vi "GetVIFolderPath.vi"(8 "error in (no error)":errorcluster, 11 "VI Reference in":refnum<vi>) -> (0 "error out":errorcluster, 3 "VI Folder Path out":path)   [LabVIEW 2015, in "VeriStandTestUtilities.lvlib"]
uses:
  VeriStandTestUtilities.lvlib
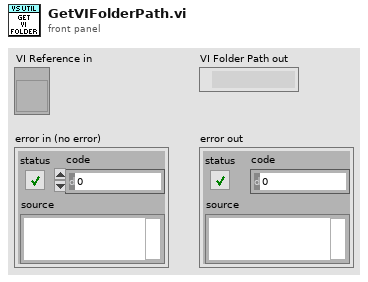
[diagram p1: front panel]
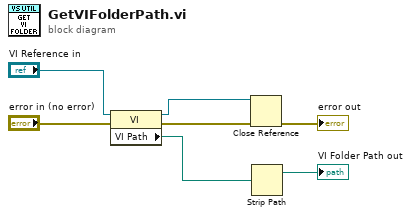
[diagram p0: block diagram]
diagram:
  n1 = property class="VI"(reference="VI Reference in", error in="error in (no error)") -> (reference out=w2:refnum<vi>, error out=w3:errorcluster, "VI Path"=w7:path)
  n2 = Close Reference(reference=w2, error in (no error)=w3) -> (error out=→"error out":errorcluster)
  n3 = Strip Path(path=w7) -> (stripped path=→"VI Folder Path out":path)  [unwired: 1 out]
